vi "VerifyArguments.vi"(8 "error in (no error)":errorcluster, 11 "RunVIAnalyzer in":refnum<class "RunVIAnalyzer.lvclass">) -> (0 "error out":errorcluster, 3 "RunVIAnalyzer out":refnum<class "RunVIAnalyzer.lvclass">)   [LabVIEW 2014, in "RunVIAnalyzer.lvclass"]
uses:
  RunVIAnalyzer.lvclass
  RunVIAnalyzer.lvclass/RunVIAnalyzer.ctl
  Utilities/OperationErrorType.ctl
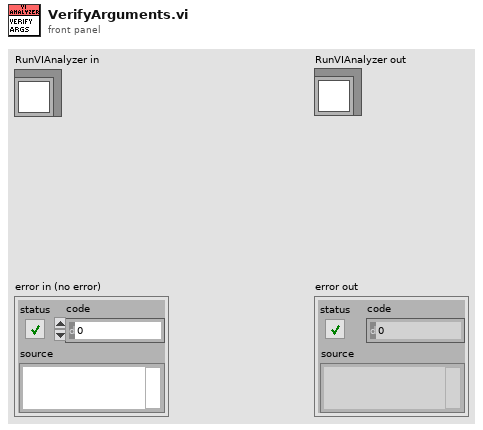
[diagram p1: front panel]
types:
  T1 = typedef "OperationErrorType.ctl" = enum16{"RequiredArgumentMissing", "UnknownArguments", "LoggerSetMultipleTimes", "OperationBrokenError"}
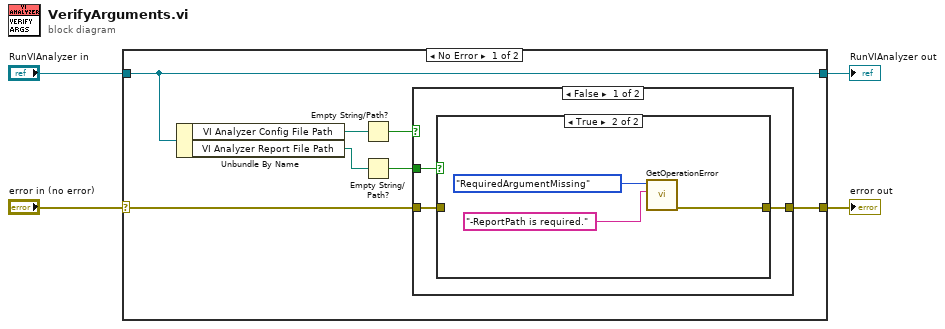
[diagram p0: block diagram]
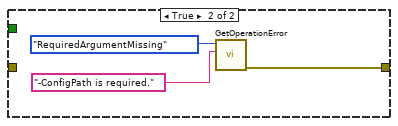
[diagram p3: hidden frame]
diagram:
  n1 = case shown="No Error" "error in (no error)" {
    selector: "error in (no error)" -> [w7 w23]
    tunnel: [w8 w23] -> w1
    tunnel: "RunVIAnalyzer in" -> [w11 w22]
    tunnel: [w11 w22] -> w2
    frame No Error {
      n2 = Unbundle By Name(w11) -> ("VI Analyzer Config File Path"=w10:path, "VI Analyzer Report File Path"=w9:path)
      n3 = Empty String/Path?(string/path=w10) -> (empty?=w6:bool)
      n4 = Empty String/Path?(string/path=w9) -> (empty?=w5:bool)
      n5 = case shown="False" w6 {
        tunnel: [w13 w19] -> w8
        tunnel: w7 -> [w12 _]
        tunnel: w5 -> [w14 _]
        frame False {
          n6 = case shown="True" w14 {
            tunnel: [w15 w18] -> w13
            tunnel: w12 -> [w15 _]
            frame False {
            }
            frame True {
              n7 = call "GetOperationError.vi"("Additional Information"="-ReportPath is required.", "Operation Error Type"=OperationErrorType."RequiredArgumentMissing") -> ("error out"=w18:errorcluster)  [unwired: 9 in]
            }
          }
        }
        frame True {
          n8 = call "GetOperationError.vi"("Additional Information"="-ConfigPath is required.", "Operation Error Type"=OperationErrorType."RequiredArgumentMissing") -> ("error out"=w19:errorcluster)  [unwired: 9 in]
        }
      }
    }
    frame Error {
    }
  }
  "error out" <- w1
  "RunVIAnalyzer out" <- w2
